vi "mass_flow_rate.vi"(1 "Density":dbl[](array[numeric]), 2 "dP Pa":dbl[](array[numeric])) -> (0 "Mass Flow Rate [g/s] Array":dbl[](array[numeric]))   [LabVIEW 2017]
uses:
  Sensor Translation/pressure_unit_converter.vi
  Sensor Translation/sensor_translation.lvlib
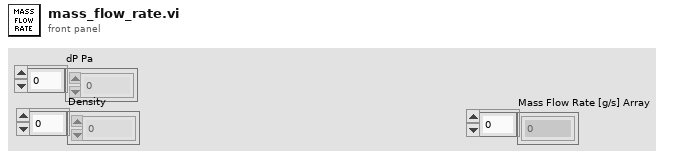
[diagram p1: front panel]
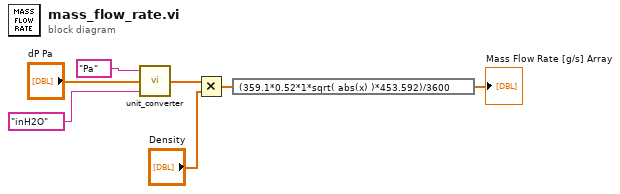
[diagram p0: block diagram]
diagram:
  n1 = call-poly "unit_converter.vi"("Output Unit"="inH2O", "Input"="dP Pa", "Input Unit"="Pa") -> ("Output"=w1:dbl[])
  n2 = Multiply(x=w1, y="Density") -> (x*y=w6:dbl[])
  n3 = expression code="(359.1*0.52*1*sqrt( abs(x) )*453.592)/3600"(w6) -> (→"Mass Flow Rate [g/s] Array":dbl[])
